vi "Division of Polynomials (DBL).vi"(9 "q":dbl[](array[numeric]), 11 "p":dbl[](array[numeric])) -> (1 "rest":dbl[](array[numeric]), 3 "p/q":dbl[](array[numeric]))   [LabVIEW 2018, in "NI_AALPro.lvlib"]
uses:
  NI_AALPro.lvlib
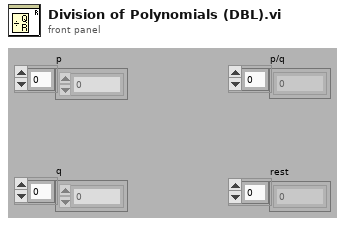
[diagram p1: front panel]
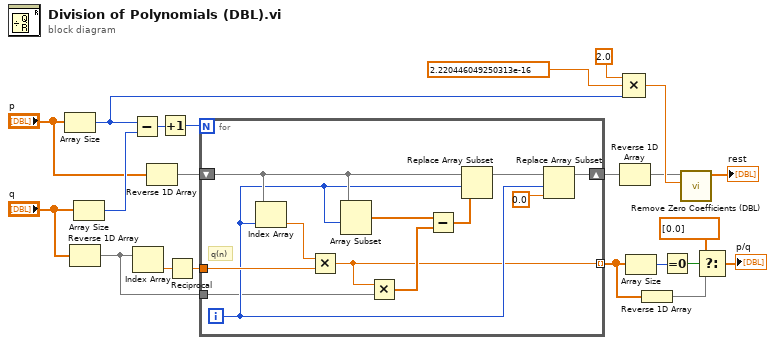
[diagram p0: block diagram]
diagram:
  n1 = Array Size(array="p") -> (size(s)=w12:i32)
  n2 = Reverse 1D Array(array="q") -> (reversed array=w5:dbl[])
  n3 = Array Size(array="q") -> (size(s)=w20:i32)
  n4 = Subtract(x=w12, y=w20) -> (x-y=w22:i32)
  n5 = Index Array(array=w5) -> (element=w2:dbl)  [unwired: 1 in]
  n6 = Reverse 1D Array(array="p") -> (reversed array=w6:dbl[])
  n7 = Increment(x=w22) -> (x+1=w21:i32)
  n8 = Reciprocal(x=w2) -> (1/x=w1:dbl)
  n9 = for {
    N: w21 -> [_]
    shift-right: [w26] -> w4
    shift-left: w6 -> [w31]
    tunnel: w5 -> [w23]
    tunnel: w1 -> [w33]
    tunnel: [w24] -> w7 mode=indexing
    i -> [w27]
    # "q(n)"
    n10 = Index Array(array=w31, index=w27) -> (element=w34:dbl)
    n11 = Multiply(x=w34, y=w33) -> (x*y=w24:dbl)
    n12 = Array Subset(array=w31, index=w27) -> (w28:dbl[])  [unwired: 1 in]
    n13 = Multiply(x=w24, y=w23) -> (x*y=w32:dbl[])
    n14 = Subtract(x=w28, y=w32) -> (x-y=w30:dbl[])
    n15 = Replace Array Subset(array=w31, new element=w30, index=w27) -> (w25:dbl[])
    n16 = Replace Array Subset(array=w25, new element=0.0 ("new element/subarray"), index=w27) -> (w26:dbl[])
  }
  n17 = Reverse 1D Array(array=w4) -> (reversed array=w3:dbl[])
  n18 = Compound Arithmetic op=MULTIPLY(2.0, 2.220446049250313e-16 ("eps for remove zeros"), w12) -> (w9:dbl)
  n19 = Array Size(array=w7) -> (size(s)=w17:i32)
  n20 = Reverse 1D Array(array=w7) -> (reversed array=w15:dbl[])
  n21 = Equal To 0?(x=w17) -> (x = 0?=w16:bool)
  n22 = call "Remove Zero Coefficients (DBL).vi"("threshold"=w9, "P(x) In"=w3) -> ("P(x) Out"=→"rest":dbl[])  [unwired: 7 in, 2 out]
  n23 = Select(t=dbl[] [0.0], s=w16, f=w15) -> (s? t:f=→"p/q":dbl[])
